vi "FGV SysLog cRIO.vi"(6 "Aktion":enum16{"initialisieren", "lesen", "schreiben"}(ring), 7 "SysLogLevel":u32, 8 "Fehler (in)":errorcluster caption="Fehler in", 10 "intern":bool, 11 "Message in":string) -> (0 "Fehler (out)":errorcluster caption="Fehlerkonstante", 1 "Fehler Array  out":errorcluster[](array[cluster]), 3 "Message out":string[](array[string]))   [LabVIEW 2020, in "SysLog_cRIO.lvlib"]
doc: "FGV zum Sammeln von Error Meldungen die mit den Betriebsdaten in eine\n#ErrLogHistory geschreiben werden - Steuerungsebene\ninitialisieren ... erzeugt ein Array (auch zum Zurücksetzen)\nspeichern ... zum Hinzufügen einer neuen Fehlermeldung\nlesen ... zum auslesen des Arrays \n\nriw 11.6.2018"
uses:
  SysLog_cRIO.lvlib
  <vilib>/regexp/Match Regular Expression.xnode
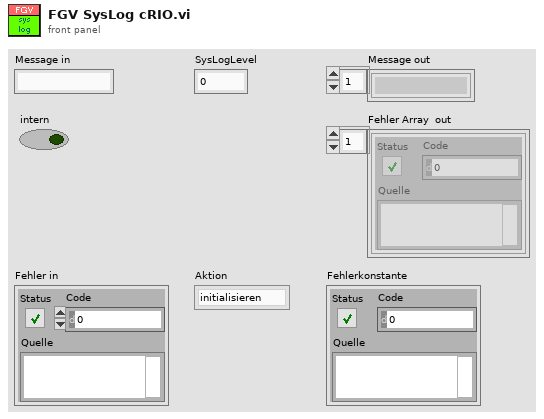
[diagram p1: front panel]
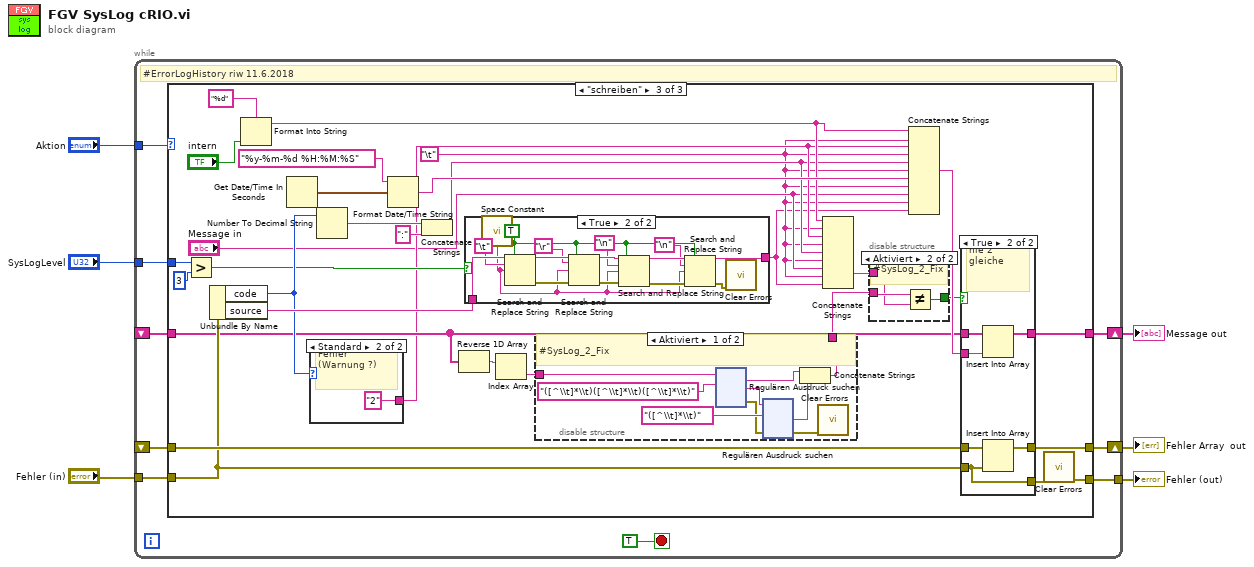
[diagram p0: block diagram]
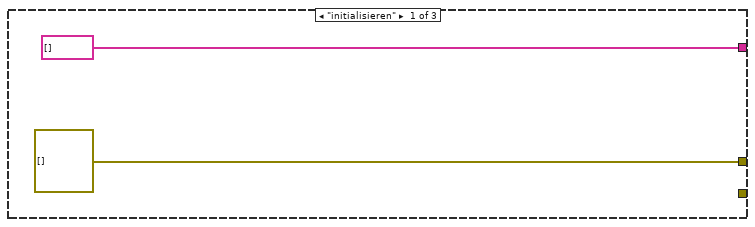
[diagram p2: hidden frame]
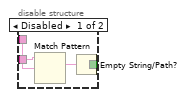
[diagram p4: hidden frame]
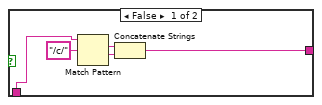
[diagram p7: hidden frame]
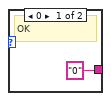
[diagram p8: hidden frame]
diagram:
  n1 = while {
    tunnel: "Aktion" -> [w15]
    shift-right: [w14] -> w4
    shift-left: _ -> [w13]
    shift-right: [w12] -> w5
    shift-left: _ -> [w11]
    tunnel: [w9] -> w3
    tunnel: "SysLogLevel" -> [w8]
    tunnel: "Fehler (in)" -> [w7]
    stop <- TRUE stop-if-true
    # "#ErrorLogHistory riw 11.6.2018"
    n2 = case shown="\"schreiben\"" w15 {
      tunnel: [errorcluster[] [] w19 w50] -> w14
      tunnel: w13 -> [_ w19 w49]
      tunnel: [string[] [] w18 w48] -> w12
      tunnel: w11 -> [_ w18 w33]
      tunnel: [_ _ w39] -> w9
      tunnel: w8 -> [_ _ w38]
      tunnel: w7 -> [_ _ w35]
      frame "initialisieren" {
      }
      frame "lesen", Default {
      }
      frame "schreiben" {
        w21 = "\t"
        n3 = Greater?(x=w38, y=u32 3) -> (0:w36:bool)
        n4 = Unbundle By Name(w35) -> ("code"=w40:i32, "source"=w43:string)
        n5 = Format Into String(format string="%d" ("Format-String"), "intern") -> (resulting string=w25:string)  [unwired: 2 in, 1 out]
        n6 = Get Date/Time In Seconds() -> (seconds since 1Jan1904=w47:timestamp)
        n7 = case shown="Standard" w40 {
          tunnel: ["0" "2"] -> w24
          frame 0 {
            # "OK"
          }
          frame Default {
            # "Fehler (Warnung ?)"
          }
        }
        n8 = Number To Decimal String(number=w40) -> (decimal integer string=w44:string)  [unwired: 1 in]
        n9 = Format Date/Time String(time format string (%c)="%y-%m-%d %H:%M:%S" ("Zeitformatierungs-String (%c)"), seconds (now)=w47) -> (date/time string=w45:string)  [unwired: 1 in]
        n10 = Concatenate Strings(w44, ":") -> (w23:string)
        n11 = Reverse 1D Array(array=w33) -> (reversed array=w31:string[])
        n12 = case shown="True" w36 {
          tunnel: w43 -> [w306 w324]
          tunnel: [w305 w316] -> w20
          frame False {
            n13 = Match Pattern(string=w306, regular expression="/c/") -> (match substring=w308:string, after substring=w307:string)  [unwired: 1 in, 2 out]
            n14 = Concatenate Strings(w308, w307) -> (w305:string)
          }
          frame True {
            w310 = TRUE ("Alle ersetzen? (F)")
            n15 = call <vilib>:"Space Constant.vi"() -> ("String"=w311:string)
            n16 = Search and Replace String(replace all?=w310, input string=w324, search string="\t", replace string=w311) -> (result string=w322:string, error out=w321:errorcluster)  [unwired: 4 in, 2 out]
            n17 = Search and Replace String(replace all?=w310, input string=w322, search string="\r", replace string=w311, error in=w321) -> (result string=w319:string, error out=w315:errorcluster)  [unwired: 3 in, 2 out]
            n18 = Search and Replace String(replace all?=w310, input string=w319, search string="\n", replace string=w311, error in=w315) -> (result string=w317:string, error out=w314:errorcluster)  [unwired: 3 in, 2 out]
            n19 = Search and Replace String(replace all?=w310, input string=w317, search string="\n", replace string=w311, error in=w314) -> (result string=w316:string, error out=w313:errorcluster)  [unwired: 3 in, 2 out]
            n20 = call <vilib>:"Clear Errors.vi"("error in (no error)"=w313) -> ()  [unwired: 5 in, 2 out]
          }
        }
        n21 = Index Array(array=w31) -> (element=w28:string)  [unwired: 1 in]
        n22 = disable-structure shown="Aktiviert" {
          disable-tunnel: w28 -> [w66 w295]
          disable-tunnel: [w59 w295] -> w27
          frame Enabled {
            # "#SysLog_2_Fix"
            n23 = xnode "Regulären Ausdruck suchen"("Eingangs-String"=w66, "Regulärer Ausdruck"="([^\\t]*\\t)([^\\t]*\\t)([^\\t]*\\t)") -> ("Komplette Übereinstimmung"=w58:string, "Nach Übereinstimmung"=w64:string, "Fehler (Ausgang)"=w62:errorcluster)  [unwired: 4 in, 2 out]
            n24 = xnode "Regulären Ausdruck suchen"("Eingangs-String"=w64, "Regulärer Ausdruck"="([^\\t]*\\t)", "Fehler (Eingang)"=w62) -> ("Nach Übereinstimmung"=w60:string, "Fehler (Ausgang)"=w61:errorcluster)  [unwired: 3 in, 3 out]
            n25 = Concatenate Strings(w58, w60) -> (w59:string)
            n26 = call <vilib>:"Clear Errors.vi"("error in (no error)"=w61) -> ()  [unwired: 5 in, 2 out]
          }
          frame Disabled {
          }
        }
        n27 = Concatenate Strings(w25, w21, w24, w21, w23, w21, "Message in", w21, w20) -> (w26:string)
        n28 = disable-structure shown="Aktiviert" {
          disable-tunnel: w26 -> [w53 w55]
          disable-tunnel: [w52 w57] -> w32
          disable-tunnel: w27 -> [w51 w56]
          frame Disabled {
            n29 = Match Pattern(string=w51, regular expression=w53) -> (match substring=w54:string)  [unwired: 1 in, 3 out]
            n30 = Empty String/Path?(string/path=w54) -> (empty?=w52:bool)
          }
          frame Enabled {
            # "#SysLog_2_Fix"
            n31 = Not Equal?(x=w56, y=w55) -> (x != y?=w57:bool)
          }
        }
        n32 = Concatenate Strings(w25, w21, w24, w21, w23, w21, w45, w21, "Message in", w21, w20) -> (w42:string)
        n33 = case shown="True" w32 {
          tunnel: [w297 w304] -> w50
          tunnel: w49 -> [w297 w303]
          tunnel: [w298 w302] -> w48
          tunnel: w33 -> [w298 w301]
          tunnel: w42 -> [_ w300]
          tunnel: w35 -> [w296 w299]
          tunnel: [w296 w299] -> w34
          frame False {
          }
          frame True {
            # "nie 2 gleiche"
            n34 = Insert Into Array(array=w301, new element=w300) -> (w302:string[])  [unwired: 1 in]
            n35 = Insert Into Array(array=w303, new element=w299) -> (w304:errorcluster[])  [unwired: 1 in]
          }
        }
        n36 = call <vilib>:"Clear Errors.vi"("error in (no error)"=w34) -> ("error out"=w39:errorcluster)  [unwired: 5 in, 1 out]
      }
    }
  }
  "Message out" <- w5
  "Fehler Array  out" <- w4
  "Fehler (out)" <- w3
